vi "报警信息通用.vi"(8 "error in (no error)":errorcluster, 10 "报警信息":string, 11 "设备":string="环境动力") -> (0 "error out":errorcluster)   [LabVIEW 2016, in "环境动力监测库.lvlib"]
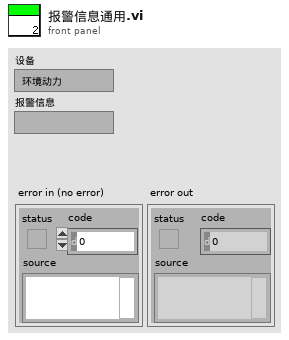
[diagram p1: front panel]
types:
  T1 = typedef "报警信息字段定义.ctl" = cluster{"时间":timestamp, "参数":string, "报警信息":string, "备注":string}
  T2 = typedef "数据库类型.ctl" = enum16{"Access", "SQLite"}
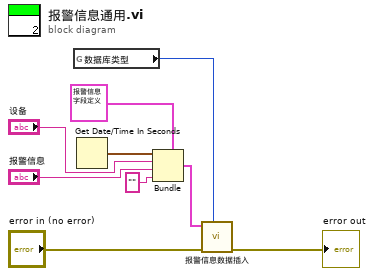
[diagram p0: block diagram]
diagram:
  n1 = global read "断电保存全局变量.vi" "数据库类型"() -> (w1:T2)
  n2 = Get Date/Time In Seconds() -> (seconds since 1Jan1904=w9:timestamp)
  n3 = Bundle(cluster=T1 {"时间"=timestamp(0 s since 1904-01-01), "参数"="水样测试", "报警信息"="N", "备注"=""} ("data"), "时间"=w9, "参数"="设备", "报警信息"="报警信息", "备注"="") -> (w4:T1)
  n4 = call "报警信息数据插入.vi"("data"=w4, "错误输入（无错误）"="error in (no error)", "数据库类型"=w1) -> ("错误输出"=→"error out":errorcluster)  [unwired: 7 in]
